vi "ReadArray.vi"(8 "error in (no error)":errorcluster, 11 "VISA resource name":refnum<visa-resource-name>) -> (0 "error out":errorcluster, 1 "Resistance (ohm)":dbl[](array[numeric]), 2 "appended array":sgl[][](array[numeric]), 3 "VISA resource name out":refnum<visa-resource-name>)   [LabVIEW 2020, in "SMU.lvclass"]
uses:
  SMU.lvclass
  <instrlib>/Keithley 24XX/Public/Data/Read (Multiple Points).vi
  <instrlib>/Keithley 24XX/Keithley 24XX.lvlib
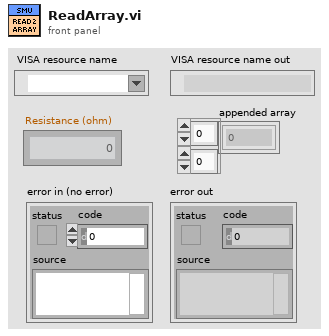
[diagram p1: front panel]
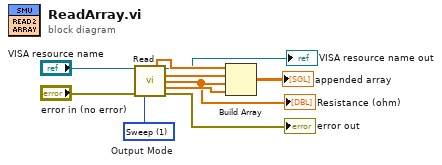
[diagram p0: block diagram]
diagram:
  w8 = u16 1 items=["Fixed", "Sweep", "List"]  # Output Mode
  n1 = call-poly <instrlib>:"Read.vi"("VISA resource name"="VISA resource name", "error in (no error)"="error in (no error)", "Output Mode (0: Fixed)"=w8) -> ("Voltage"=w3:sgl[], "VISA resource name out"=→"VISA resource name out":refnum<visa-resource-name>, "Current"=w7:sgl[], "Resistance"=w1:sgl[], "Timestamp"=w10:sgl[], "error out"=→"error out":errorcluster)  [unwired: 6 in, 1 out]
  "Resistance (ohm)" <- w1
  n2 = Build Array(w3, w7, w1, w10) -> (→"appended array":sgl[][])
